vi "Create Background Colors.vi"(10 "iItem names":string[](array[string]), 11 "change flag":bool) -> (2 "background colors":u32[](array[colorbox]))   [LabVIEW 2020, in "Ballard ARINC 429 System Explorer.lvlib" / "Implementation.lvlib"]
doc: "This VI runs when the Add Port run-time menu is chosen. It allows the user to create a port with an associated database."
uses:
  Implementation.lvlib
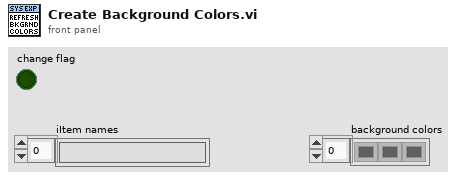
[diagram p1: front panel]
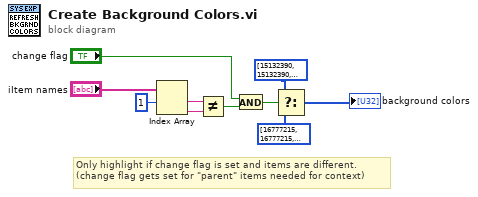
[diagram p0: block diagram]
diagram:
  # "Only highlight if change flag is set and items are different.\n(change flag gets set for \"parent\" items needed for context)"
  n1 = Index Array(array="iItem names", index #1=1 ("index")) -> (element #1=w6:string, element #2=w7:string)  [unwired: 1 in]
  n2 = Not Equal?(x=w6, y=w7) -> (x != y?=w5:bool)
  n3 = And(x="change flag", y=w5) -> (x .and. y?=w4:bool)
  n4 = Select(t=u32[] [15132390, 15132390, 15132390] ("Bulk Cells:Background Colors"), s=w4, f=u32[] [16777215, 16777215, 16777215] ("Bulk Cells:Background Colors")) -> (s? t:f=→"background colors":u32[])
